vi "AGCxxx Query GAuge.vi"(8 "error in (no error)":errorcluster, 10 "Channel (0)":i32, 11 "AGCxxx VISA Cluster":T1={"VISA resource name"="", "VISA Timeout Value (1000 ms)"=1000, "Lock Timeout (1000 ms)"=1000, "MAX Channel (6)"=6}) -> (0 "error out":errorcluster, 1 "AGC Errno":i32, 2 "Gauge":dbl format="%.4e", 3 "dup AGCxxx VISA Cluster":T1={"VISA resource name"="", "VISA Timeout Value (1000 ms)"=1000, "Lock Timeout (1000 ms)"=1000, "MAX Channel (6)"=6})   [LabVIEW 2014, in "AGCxxx - Driver.lvlib"]
doc: "Returns the current pressure reading for gauge channel x, as displayed on the front panel of the AGC.\nPressure displayed as mEse where m is the mantissa, s the sign + or -, and e is the exponent.\n\nCopyright (C) \nGesellschaft f. Schwerionenforschung, GSI\nPlanckstr. 1\n64291 Darmstadt\nGermany\n\nContact: http://www-wnt.gsi.de/labview\n H.Brand@gsi.de\n\nThis program is free software; you can redistribute it and/or\nmodify it under the terms of the GNU General Public License\nas published by the Free Software Foundation; either version 2\nof the License, or (at your option) any later version.\n\nThis program is distributed in the hope that it will be useful,\nbut WITHOUT ANY WARRANTY; without even the implied warranty of\nMERCHANTABILITY or FITNESS FOR A PARTICULAR PURPOSE. See the\nGNU General Public License for more details (http://www.gnu.org)."
uses:
  AGCxxx - Driver.lvlib
  AGCxxx VISA Control.ctl
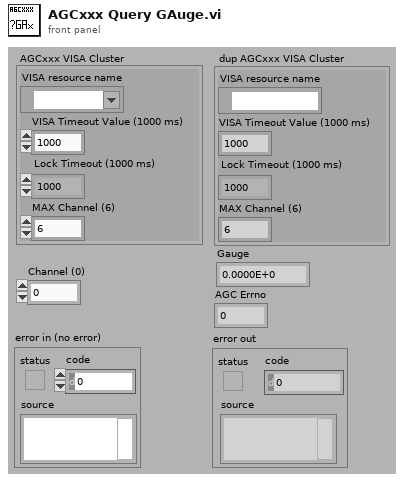
[diagram p1: front panel]
types:
  T1 = typedef "AGCxxx - Driver.lvlib/AGCxxx VISA Control.ctl" = cluster{"VISA resource name":refnum<visa-resource-name>, "VISA Timeout Value (1000 ms)":u32, "Lock Timeout (1000 ms)":u32, "MAX Channel (6)":i32}
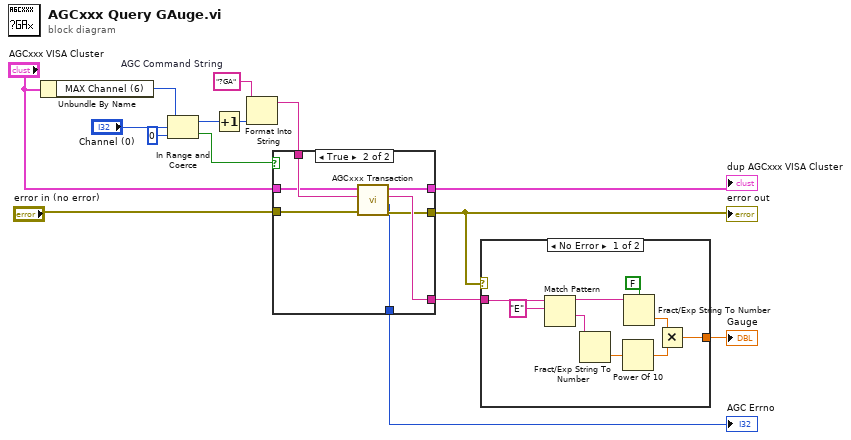
[diagram p0: block diagram]
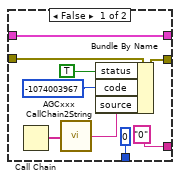
[diagram p2: hidden frame]
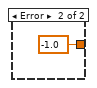
[diagram p3: hidden frame]
diagram:
  w11 = "?GA"  # AGC Command String
  n1 = Unbundle By Name("AGCxxx VISA Cluster") -> ("MAX Channel (6)"=w4:i32)
  n2 = In Range and Coerce(upper limit=w4, x="Channel (0)", lower limit=0) -> (coerced(x)=w3:i32, In Range?=w8:bool)
  n3 = Increment(x=w3) -> (x+1=w1:i32)
  n4 = Format Into String(initial string=w11, w1) -> (resulting string=w10:string)  [unwired: 2 in, 1 out]
  n5 = case shown="True" w8 {
    tunnel: ["0" ("AGC Response") w31] -> w15
    tunnel: [w19 w25] -> w5
    tunnel: [w23 w30] -> w14
    tunnel: "error in (no error)" -> [w24 w29]
    tunnel: [0 ("AGC Errno") w28] -> w12
    tunnel: w10 -> [_ w27]
    tunnel: "AGCxxx VISA Cluster" -> [w19 w26]
    frame False {
      n6 = Call Chain() -> (call chain=w18:string[])
      n7 = call "AGCxxx CallChain2String.vi"("call chain"=w18) -> ("Call Chain String"=w16:string)
      n8 = Bundle By Name(cluster=w24, "status"=TRUE, "code"=-1074003967, "source"=w16) -> (w23:errorcluster)
    }
    frame True {
      n9 = call "AGCxxx Transaction.vi"("error in (no error)"=w29, "AGC Command String"=w27, "AGCxxx VISA Cluster"=w26) -> ("error out"=w30:errorcluster, "AGC Errno"=w28:i32, "AGC Response"=w31:string, "dup AGCxxx VISA Cluster"=w25:T1)  [unwired: 4 in]
    }
  }
  "error out" <- w14
  "AGC Errno" <- w12
  "dup AGCxxx VISA Cluster" <- w5
  n10 = case shown="No Error" w14 {
    tunnel: w15 -> [w33 _]
    tunnel: [w32 -1.0] -> w2
    frame No Error {
      n11 = Match Pattern(string=w33, regular expression="E" ("search string/char (-)")) -> (before substring=w36:string, after substring=w39:string)  [unwired: 1 in, 2 out]
      n12 = Fract/Exp String To Number(string=w39) -> (number=w38:dbl)  [unwired: 3 in, 1 out]
      n13 = Power Of 10(x=w38) -> (10^x=w34:dbl)
      n14 = Fract/Exp String To Number(use system decimal point (T)=FALSE, string=w36) -> (number=w37:dbl)  [unwired: 2 in, 1 out]
      n15 = Multiply(x=w37, y=w34) -> (x*y=w32:dbl)
    }
    frame Error {
    }
  }
  "Gauge" <- w2
